vi "test.vi"() -> ()   [LabVIEW 2020]
uses:
  <vilib>/drjdpowell/SQLite Library/SQL Connection/Open (path).vi
  <vilib>/drjdpowell/SQLite Library/SQL Connection/Open (string).vi
  <vilib>/AdvancedString/Path To Command Line String.vi
  <vilib>/drjdpowell/SQLite Library/SQL Connection/Execute SQL.vi
  <vilib>/drjdpowell/SQLite Library/SQL Connection/Execute SQL (No results).vi
  <vilib>/drjdpowell/SQLite Library/SQL Connection/Connection.lvclass
  <vilib>/drjdpowell/SQLite Library/SQLite.lvlib
  <vilib>/drjdpowell/SQLite Library/Transaction Helpers/Transaction.lvlib
  <vilib>/drjdpowell/SQLite Library/SQL Statement/SQL Statement.lvclass
  <vilib>/drjdpowell/SQLite Library/SQL Connection/Execute SQL (Single DBL).vi
panel:
  out "Result Set":string[][](array[string])
  out "Result":dbl format="%.6g"
  in  "SQL":string="DROP TABLE MyTest;\nCREATE TABLE MyTest(X,Y)"
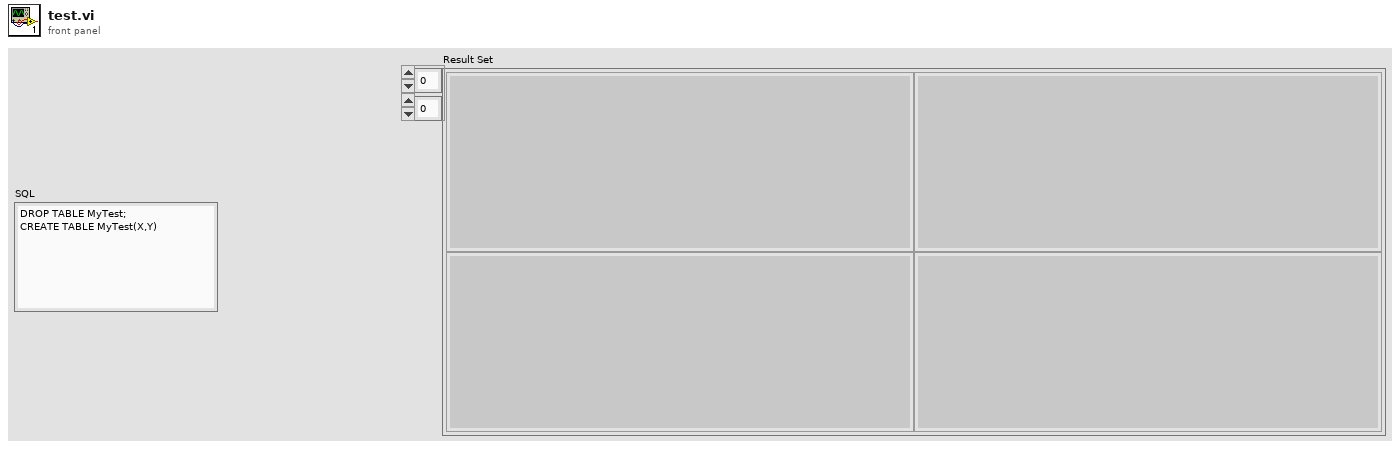
[diagram p1: front panel]
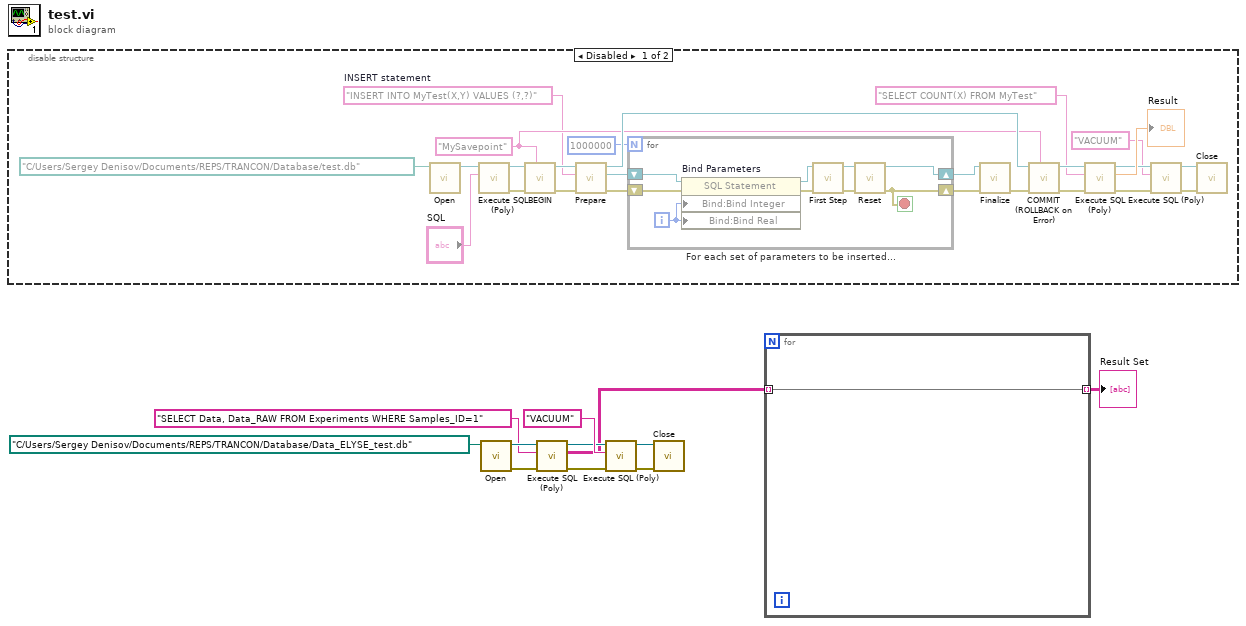
[diagram p0: block diagram]
diagram:
  n1 = disable-structure shown="Disabled" {
    frame Disabled {
      w32 = "MySavepoint" ("Savepoint name")
      w27 = "INSERT INTO MyTest(X,Y) VALUES (?,?)"  # INSERT statement
      n2 = call-poly <vilib>:"Open.vi"("db file"=path "C:/Users/Sergey Denisov/Documents/REPS/TRANCON/Database/test.db") -> ("SQLite Connection"=w12:refnum<class "Connection.lvclass">)  [unwired: 9 in, 1 out]
      n3 = call-poly <vilib>:"Execute SQL (Poly).vi"("SQL"="SQL", "SQLite Connection in"=w12) -> ("error out"=w23:errorcluster, "SQLite Connection"=w24:refnum<class "Connection.lvclass">)  [unwired: 8 in]
      n4 = call <vilib>:"BEGIN.vi"("Savepoint name"=w32, "error in (no error)"=w23, "SQLite Connection in"=w24) -> ("error out"=w31:errorcluster, "SQLite Connection"=w30:refnum<class "Connection.lvclass">)  [unwired: 7 in]
      n5 = call <vilib>:"Prepare.vi"("error in (no error)"=w31, "SQL"=w27, "SQLite Connection in"=w30) -> ("error out"=w26:errorcluster, "SQL Statement"=w25:refnum<class "SQL Statement.lvclass">, "SQLite Connection"=w33:refnum<class "Connection.lvclass">)  [unwired: 4 in, 2 out]
      n6 = for "For each set of parameters to be inserted..." {
        N: 1000000 -> [_]
        shift-right: [w39] -> w28
        shift-left: w25 -> [w45]
        shift-right: [w38] -> w29
        shift-left: w26 -> [w42]
        i -> [w37]
        stop <- w38 stop-if-true
        n7 = property on="Bind Parameters" class="SQL Statement"(reference=w45, error in=w42, "Bind:Bind Integer"=w37, "Bind:Bind Real"=w37) -> (reference out=w44:refnum<class "SQL Statement.lvclass">, error out=w43:errorcluster)
        n8 = call <vilib>:"First Step.vi"("error in (no error)"=w43, "SQL Statement in"=w44) -> ("error out"=w41:errorcluster, "SQL Statement"=w40:refnum<class "SQL Statement.lvclass">)  [unwired: 7 in, 1 out]
        n9 = call <vilib>:"Reset.vi"("error in (no error)"=w41, "SQL Statement in"=w40) -> ("error out"=w38:errorcluster, "SQL Statement"=w39:refnum<class "SQL Statement.lvclass">)  [unwired: 8 in]
      }
      n10 = call <vilib>:"Finalize.vi"("error in (no error)"=w29, "SQL Statement in"=w28) -> ("error out"=w34:errorcluster)  [unwired: 9 in]
      n11 = call <vilib>:"COMMIT (ROLLBACK on Error).vi"("Savepoint name"=w32, "error in (no error)"=w34, "SQLite Connection in"=w33) -> ("error out"=w21:errorcluster, "SQLite Connection"=w20:refnum<class "Connection.lvclass">)  [unwired: 7 in]
      n12 = call-poly <vilib>:"Execute SQL (Poly).vi"("error in (no error)"=w21, "SQL"="SELECT COUNT(X) FROM MyTest", "SQLite Connection in"=w20) -> ("error out"=w16:errorcluster, "Result"=→"Result":dbl, "SQLite Connection"=w17:refnum<class "Connection.lvclass">)  [unwired: 6 in]
      n13 = call-poly <vilib>:"Execute SQL (Poly).vi"("error in (no error)"=w16, "SQL"="VACUUM", "SQLite Connection in"=w17) -> ("error out"=w13:errorcluster, "SQLite Connection"=w14:refnum<class "Connection.lvclass">)  [unwired: 6 in, 1 out]
      n14 = call-dynamic "Close.vi"("error in (no error)"=w13, "SQLite Connection in"=w14) -> ()  [unwired: 9 in, 1 out]
    }
    frame Enabled {
    }
  }
  n15 = call-poly <vilib>:"Open.vi"("db file"=path "C:/Users/Sergey Denisov/Documents/REPS/TRANCON/Database/Data_ELYSE_test.db") -> ("error out"=w9:errorcluster, "SQLite Connection"=w10:refnum<class "Connection.lvclass">)  [unwired: 9 in]
  n16 = call-poly <vilib>:"Execute SQL (Poly).vi"("error in (no error)"=w9, "SQL"="SELECT Data, Data_RAW FROM Experiments WHERE Samples_ID=1", "SQLite Connection in"=w10) -> ("error out"=w3:errorcluster, "Result Set"=w2:string[][], "SQLite Connection"=w6:refnum<class "Connection.lvclass">)  [unwired: 5 in, 1 out]
  n17 = call-poly <vilib>:"Execute SQL (Poly).vi"("error in (no error)"=w3, "SQL"="VACUUM", "SQLite Connection in"=w6) -> ("error out"=w4:errorcluster, "SQLite Connection"=w5:refnum<class "Connection.lvclass">)  [unwired: 7 in]
  n18 = call-dynamic "Close.vi"("error in (no error)"=w4, "SQLite Connection in"=w5) -> ()  [unwired: 9 in, 1 out]
  n19 = for {
    tunnel: w2 -> [w46] mode=indexing
    tunnel: [w46] -> w1 mode=indexing
  }
  "Result Set" <- w1
